vi "Check CAN DMA.vi"(8 "error in (no error)":errorcluster, 11 "Bitfile path":path=path "\\\\vmware-host\\Shared Folders/_Repo/CAN-Frame-Protection-Custom-Device/Source/SubModules/985x-Support/Source/FPGA Bitfiles/985xsupport_FPGATarget_985x-fpga-main_Zh67qEb7W8k.lvbitx") -> (0 "error out":errorcluster, 3 "Found":bool)   [LabVIEW 2020, in "985x Support System Explorer.lvlib"]
uses:
  985x Support System Explorer.lvlib
  <vilib>/rvi/ClientSDK/Host Interface/DMA/public/niFpgaDmaChannelVisibilityFilter.ctl
  <vilib>/rvi/ClientSDK/Core/ModuleGeneration/CommunicationInterfaceUtility/niFpgaDmaChannelImplementation.ctl
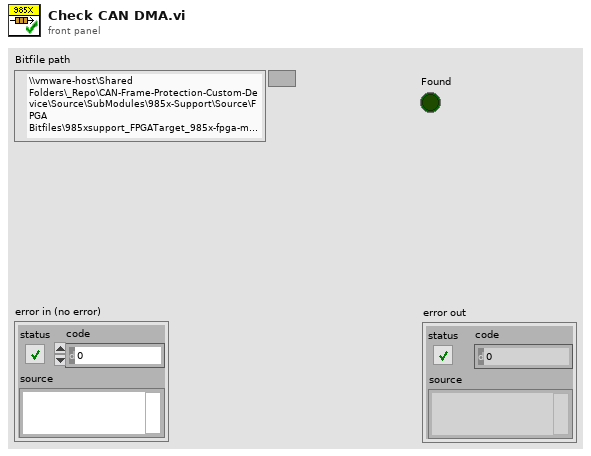
[diagram p1: front panel]
types:
  T1 = typedef "niFpgaDmaChannelVisibilityFilter.ctl" = enum16{"All", "UserVisible"}
  T2 = typedef "niFpgaDmaChannelImplementation.ctl" = enum16{"niFpgaTargetToHost", "niFpgaHostToTarget", "niFpgaPeerToPeerWriter", "niFpgaPeerToPeerReader", "niCoreTargetToHost", "niCoreHostToTarget"}
  T3 = typedef "Fifo_DMA_Config.ctl" = cluster{"Name":string, "Depth":u32, "Write? (Deprecated:Use Implementation)":bool, "Physical Channel":u32, "Base Address":u32, "Data Width":u32, "Data Type":T4, "FXP Properties":variant, "Write Window Address":u32, "Implementation":T2, "Control Set":u32}
  T4 = typedef "niFpgaDataTypeControl.ctl" = enum32{"Boolean", "I8", "I16", "I32", "I64", "U8", "U16", "U32", "U64", "FXP", "CustomControl", "SGL"}
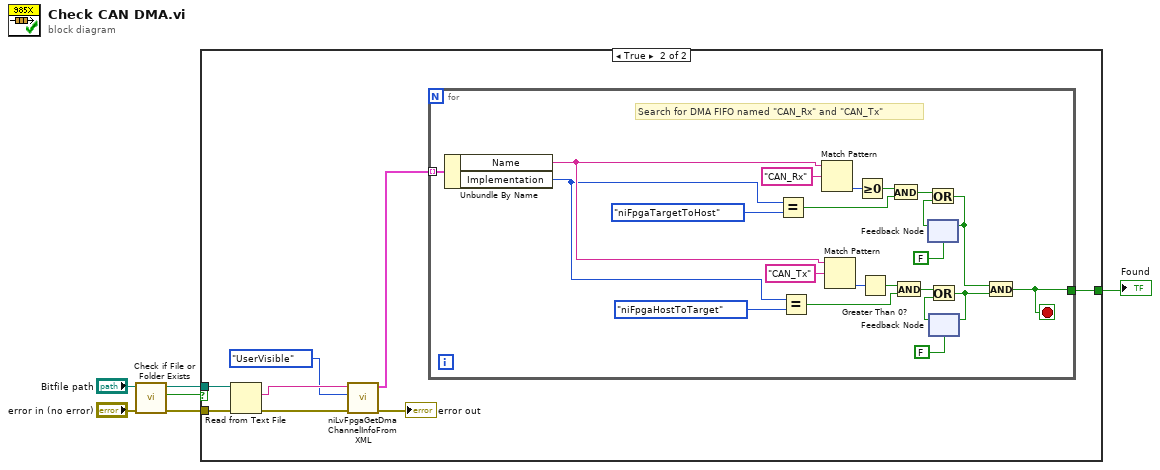
[diagram p0: block diagram]
diagram:
  n1 = call <vilib>:"Check if File or Folder Exists.vi"("error in (no error)"="error in (no error)", "path"="Bitfile path") -> ("error out"=w4:errorcluster, "file or folder exists?"=w1:bool, "dup path"=w2:path)  [unwired: 7 in]
  n2 = case shown="True" w1 {
    tunnel: w2 -> [_ w14]
    tunnel: w4 -> [_ w13]
    tunnel: [_ w7] -> w6
    frame False {
    }
    frame True {
      n3 = Read from Text File(file (use dialog)=w14, error in=w13) -> (text=w12:string, error out=w11:errorcluster)  [unwired: 2 in, 2 out]
      n4 = call <resource>:"niLvFpgaGetDmaChannelInfoFromXML.vi"("error in (no error)"=w11, "DMA Channel Filter"=niFpgaDmaChannelVisibilityFilter."UserVisible", "XML String in"=w12) -> ("error out"=→"error out":errorcluster, "DMA configuration array"=w8:T3[])  [unwired: 7 in]
      n5 = for {
        tunnel: w8 -> [w36] mode=indexing
        tunnel: [w15] -> w7
        stop <- w15 stop-if-true
        # "Search for DMA FIFO named \"CAN_Rx\" and \"CAN_Tx\""
        n6 = Unbundle By Name(w36) -> ("Name"=w26:string, "Implementation"=w25:T2)
        n7 = Equal?(x=w25, y=niFpgaDmaChannelImplementation."niFpgaTargetToHost" ("Implementation")) -> (x = y?=w32:bool)
        n8 = Equal?(x=w25, y=niFpgaDmaChannelImplementation."niFpgaHostToTarget" ("Implementation")) -> (x = y?=w27:bool)
        n9 = Match Pattern(string=w26, regular expression="CAN_Rx") -> (offset past match=w33:i32)  [unwired: 1 in, 3 out]
        n10 = Match Pattern(string=w26, regular expression="CAN_Tx") -> (offset past match=w29:i32)  [unwired: 1 in, 3 out]
        n11 = Greater Or Equal To 0?(x=w33) -> (x >= 0?=w23:bool)
        n12 = Greater Than 0?(x=w29) -> (x > 0?=w28:bool)
        n13 = And(x=w23, y=w32) -> (x .and. y?=w22:bool)
        n14 = And(x=w28, y=w27) -> (x .and. y?=w18:bool)
        n15 = feedback #1(FALSE) -> (w21:bool)
        n16 = Or(x=w22, y=w21) -> (x .or. y?=w17:bool)
        n17 = feedback-in #1(w17) -> ()
        n18 = feedback #2(FALSE) -> (w20:bool)
        n19 = Or(x=w18, y=w20) -> (x .or. y?=w16:bool)
        n20 = feedback-in #2(w16) -> ()
        n21 = And(x=w17, y=w16) -> (x .and. y?=w15:bool)
      }
    }
  }
  "Found" <- w6
